vi "Fdx Get Tx Status.vi"(8 "error in (no error)":errorcluster, 11 "InstrumentHandle_port in":u32) -> (0 "error out":errorcluster, 1 "TxStatus":T1, 3 "InstrumentHandle_port out":u32)   [LabVIEW 2020, in "AIM664LV.lvlib"]
uses:
  AIM664LV.lvlib
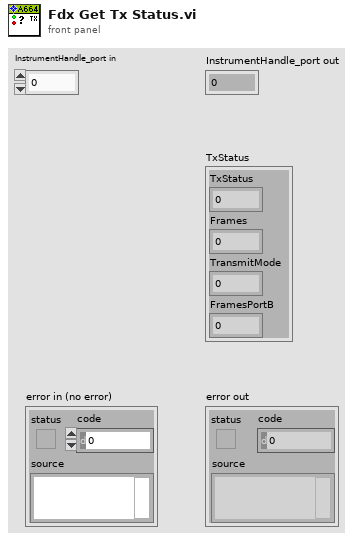
[diagram p1: front panel]
types:
  T1 = cluster{"TxStatus":u32, "Frames":u32, "TransmitMode":u32, "FramesPortB":u32}
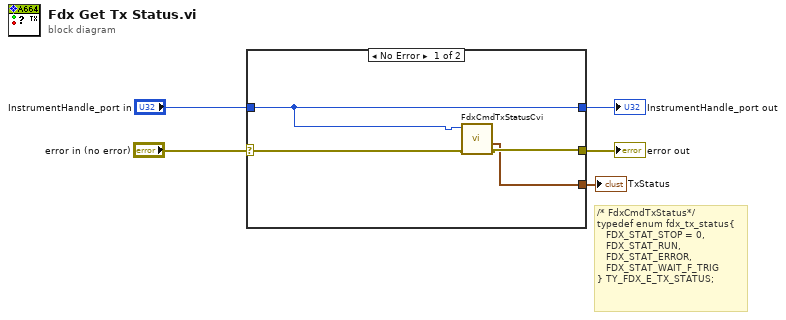
[diagram p0: block diagram]
diagram:
  # "/* FdxCmdTxStatus*/\ntypedef enum fdx_tx_status{\n   FDX_STAT_STOP = 0,\n   FDX_STAT_RUN,\n   FDX_STAT_ERROR,\n   FDX_STAT_WAIT_F_TRIG\n} TY_FDX_E_TX_STATUS;"
  n1 = case shown="No Error" "error in (no error)" {
    selector: "error in (no error)" -> [w9 w10]
    tunnel: "InstrumentHandle_port in" -> [w6 w11]
    tunnel: [w8 w10] -> w3
    tunnel: [w6 w11] -> w2
    tunnel: [w7 _] -> w1
    frame No Error {
      n2 = call "FdxCmdTxStatusCvi.vi"("error in"=w9, "InstrumentHandle_port"=w6) -> ("error out"=w8:errorcluster, "TxStatus"=w7:T1)  [unwired: 7 in, 1 out]
    }
    frame Error {
    }
  }
  "error out" <- w3
  "InstrumentHandle_port out" <- w2
  "TxStatus" <- w1
